vi "PS4000_stream.vi"() -> ()   [LabVIEW 2009]
uses:
  PS4000.dll
  ps4000wrap.dll
  Instance           1 21Saved   PS4000_stream .vi
panel:
  out "Sampling Interval (nanoseconds)":i32
  in  "Number of samples":i32
  in  "Sample Rate (S/s)":u32
  out "bufferLth":i32
  out "Triggered":bool
  in  "Threshold (mV)":i16
  in  "Auto Trigger (ms)":i32 min=1
  in  "Trigger direction":i16(ring) items=["Rising", "Falling"]
  in  "Update settings":bool
  in  "Ch A Coupling":enum32{"Radio Selection 1", "Radio Selection 2"}(radio)
  in  "Ch B Coupling":enum32{"Radio Selection 1", "Radio Selection 2"}(radio)
  out "XY Graph":cluster{"buffer":dbl[], "buffer":dbl[]}(graph)
  in  "Trigger delay (us)":u32
  in  "Ch A Trigger":bool
  in  "A enabled":bool
  in  "B enabled":bool
  out "Channel B":waveform(dbl)(graph)
  in  "Ch B Range":i32(ring) items=["±50 mV", "±100 mV", "±200 mV", "±500 mV", "±1 V", "±2 V", "±5 V", "±10 V", "±20 V", "±50 V", "±100 V"]
  in  "Ch A Range":i32(ring) items=["±50 mV", "±100 mV", "±200 mV", "±500 mV", "±1 V", "±2 V", "±5 V", "±10 V", "±20 V", "±50 V", "±100 V"]
  in  "stop":bool
  out "Channel A":waveform(dbl)(graph)
  # "Streaming example"
  # "(Must be within channel range)"
  # "X-Y Plot"
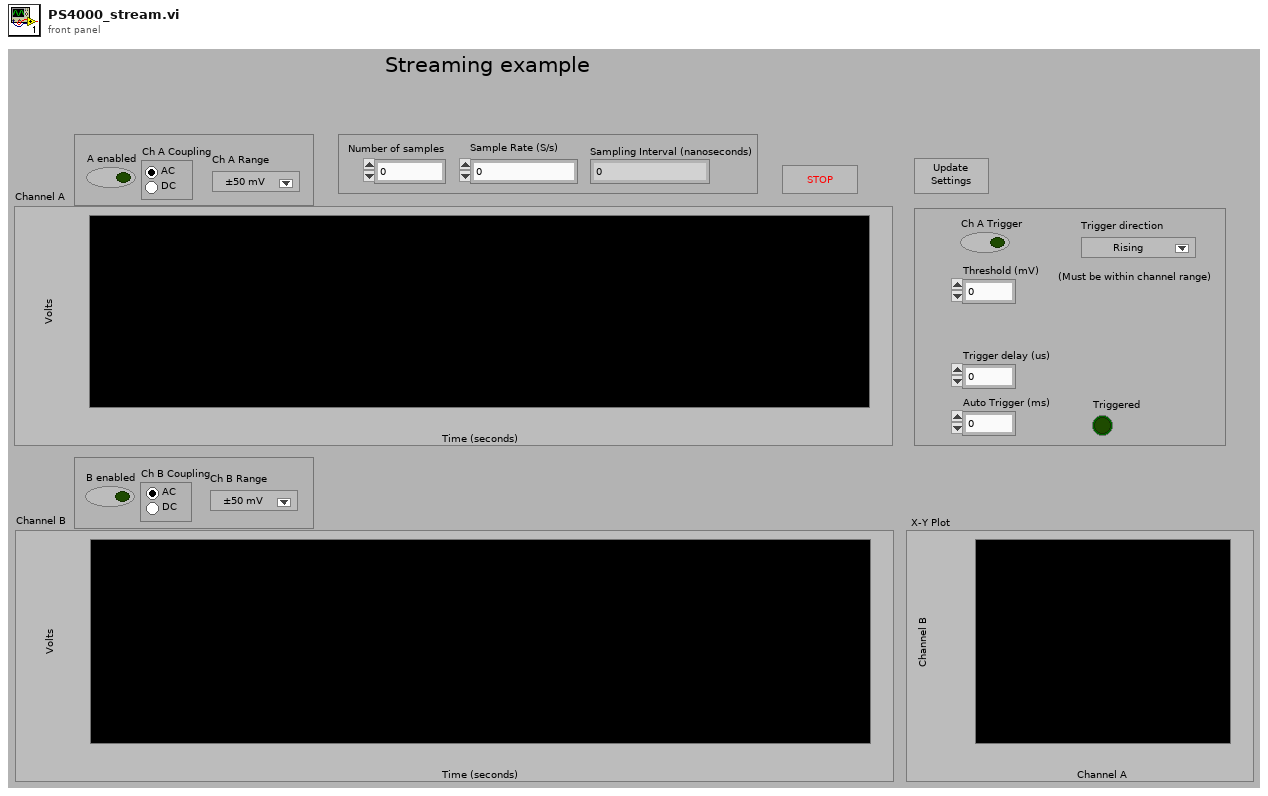
[diagram p1: front panel]
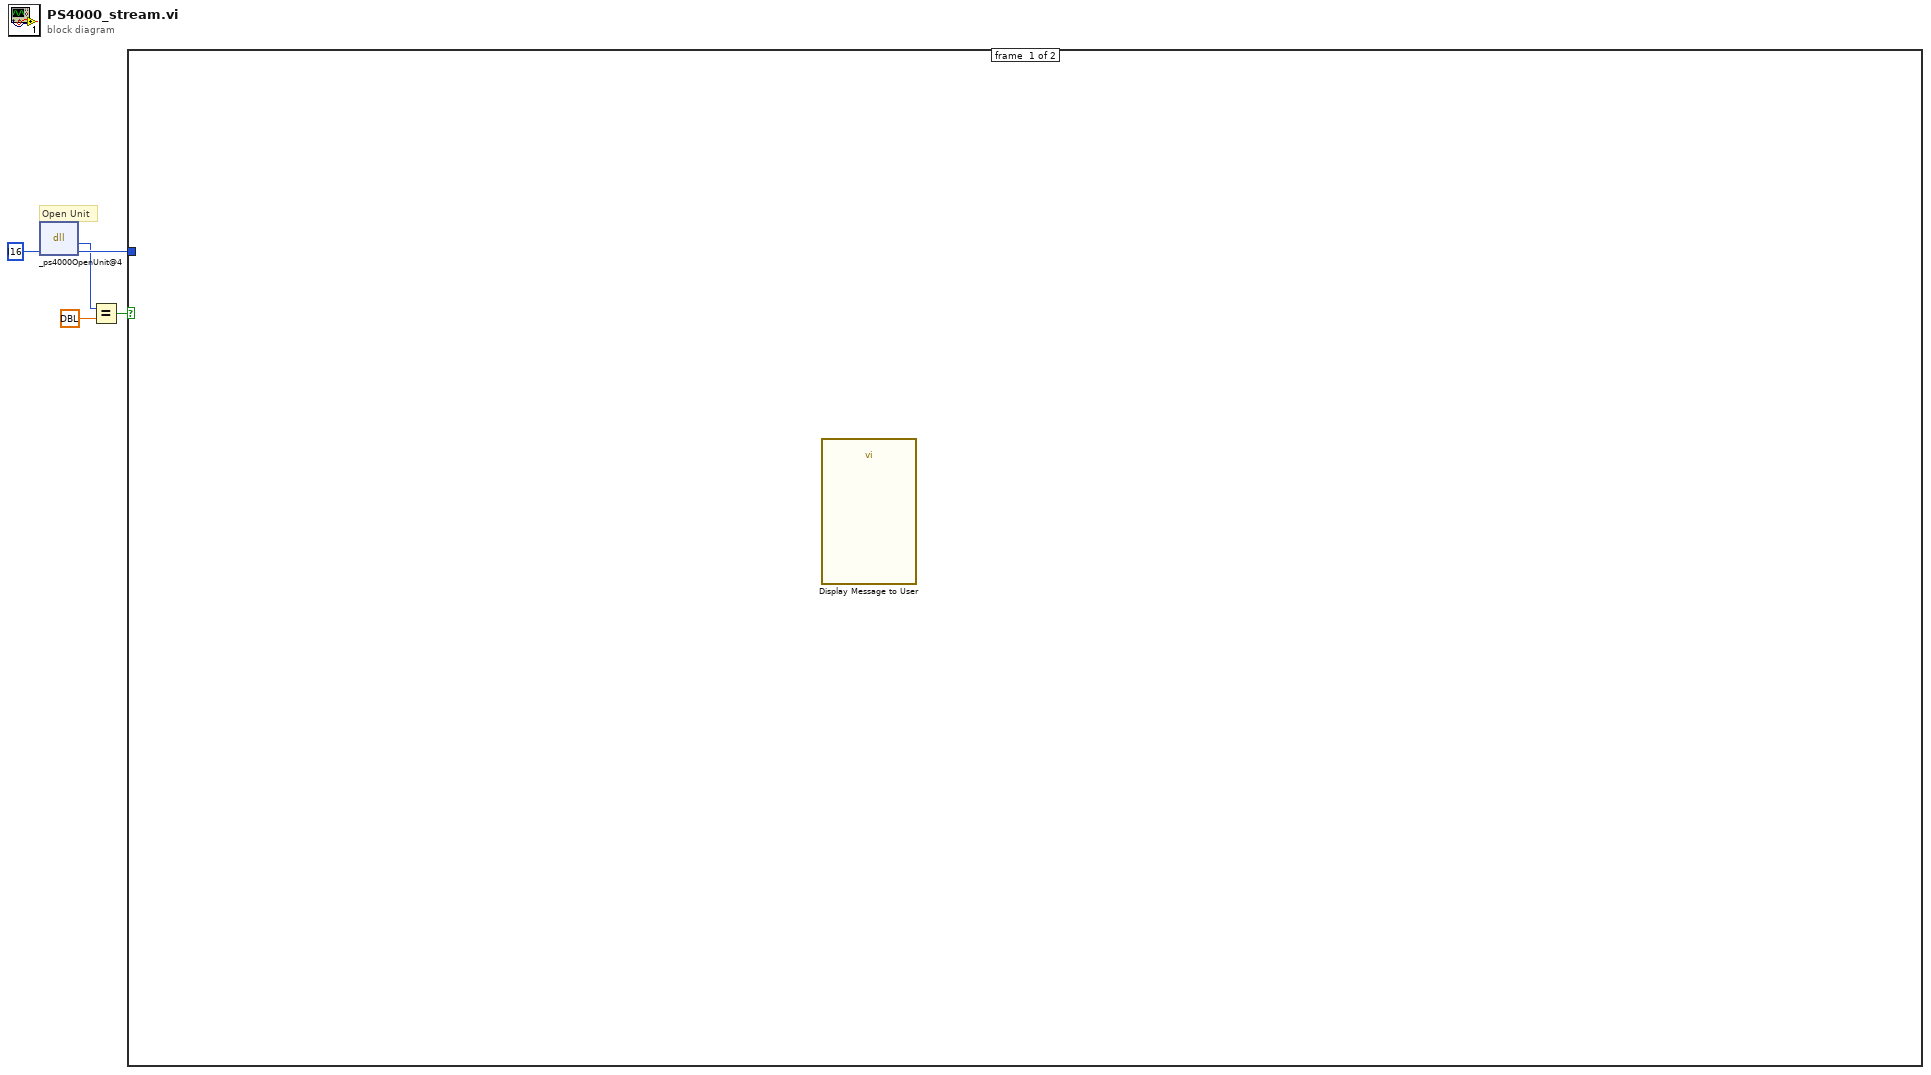
[diagram p0: block diagram]
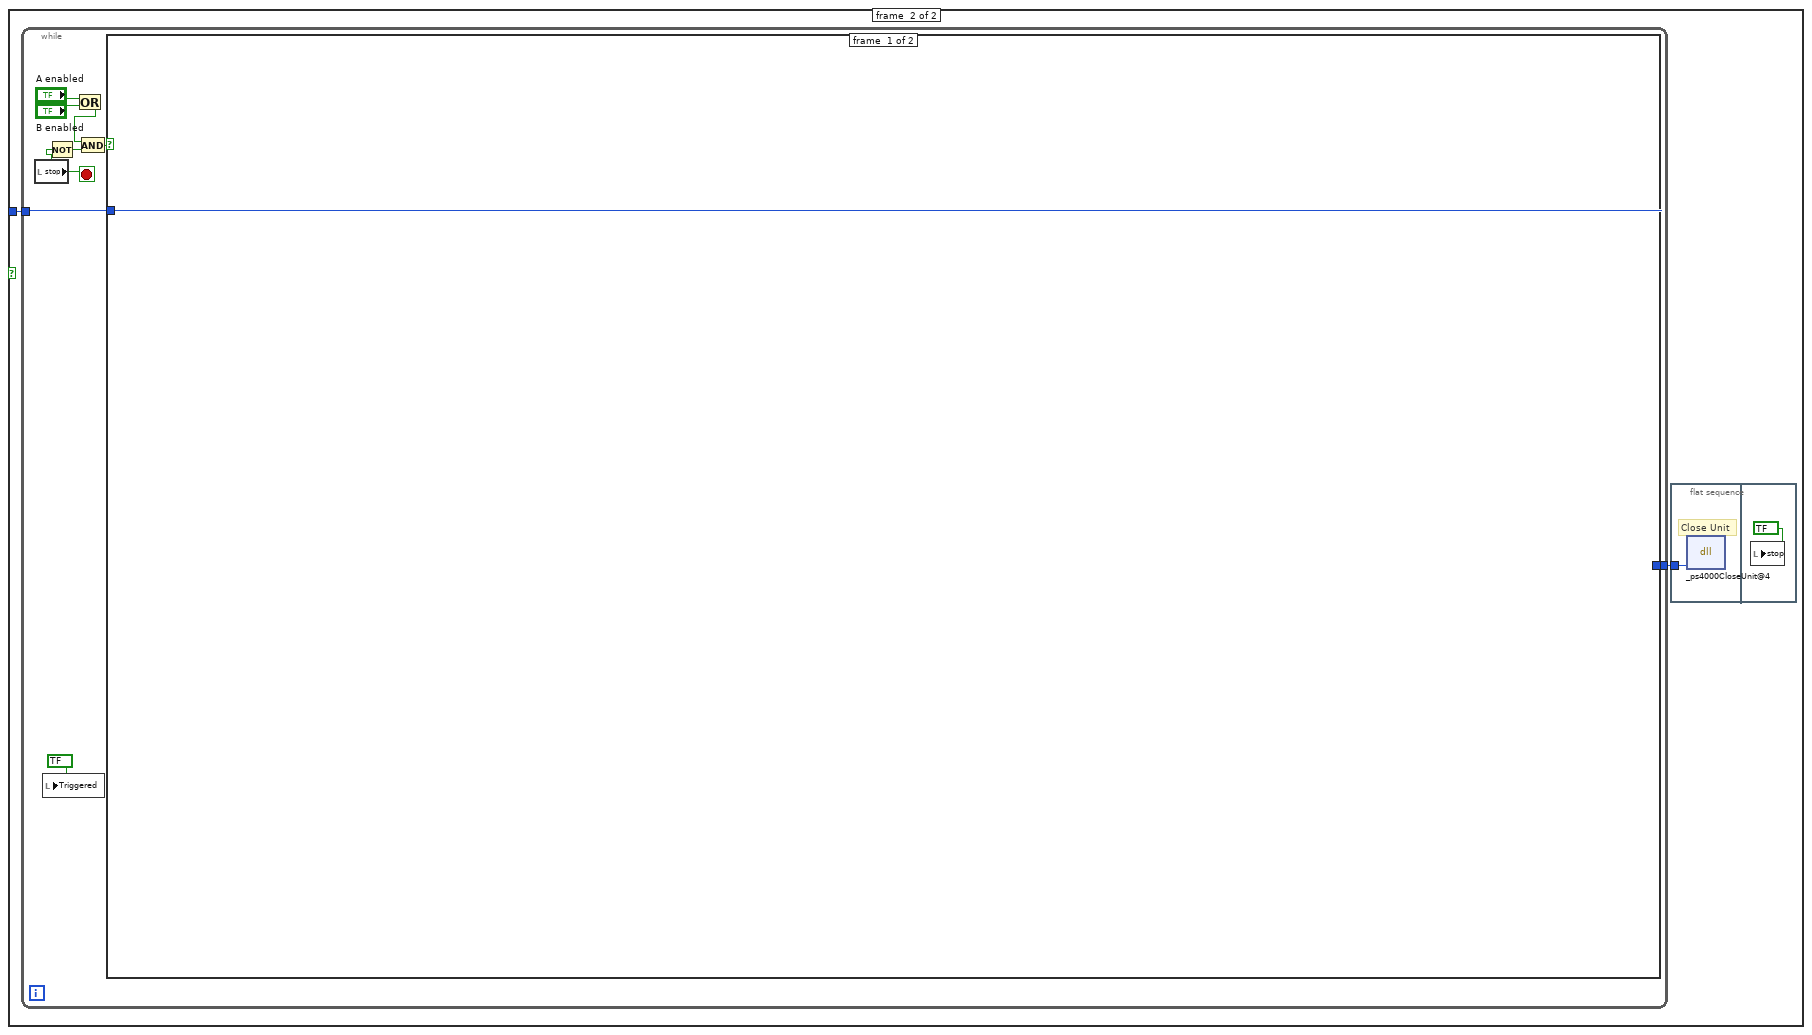
[diagram p2: hidden frame]
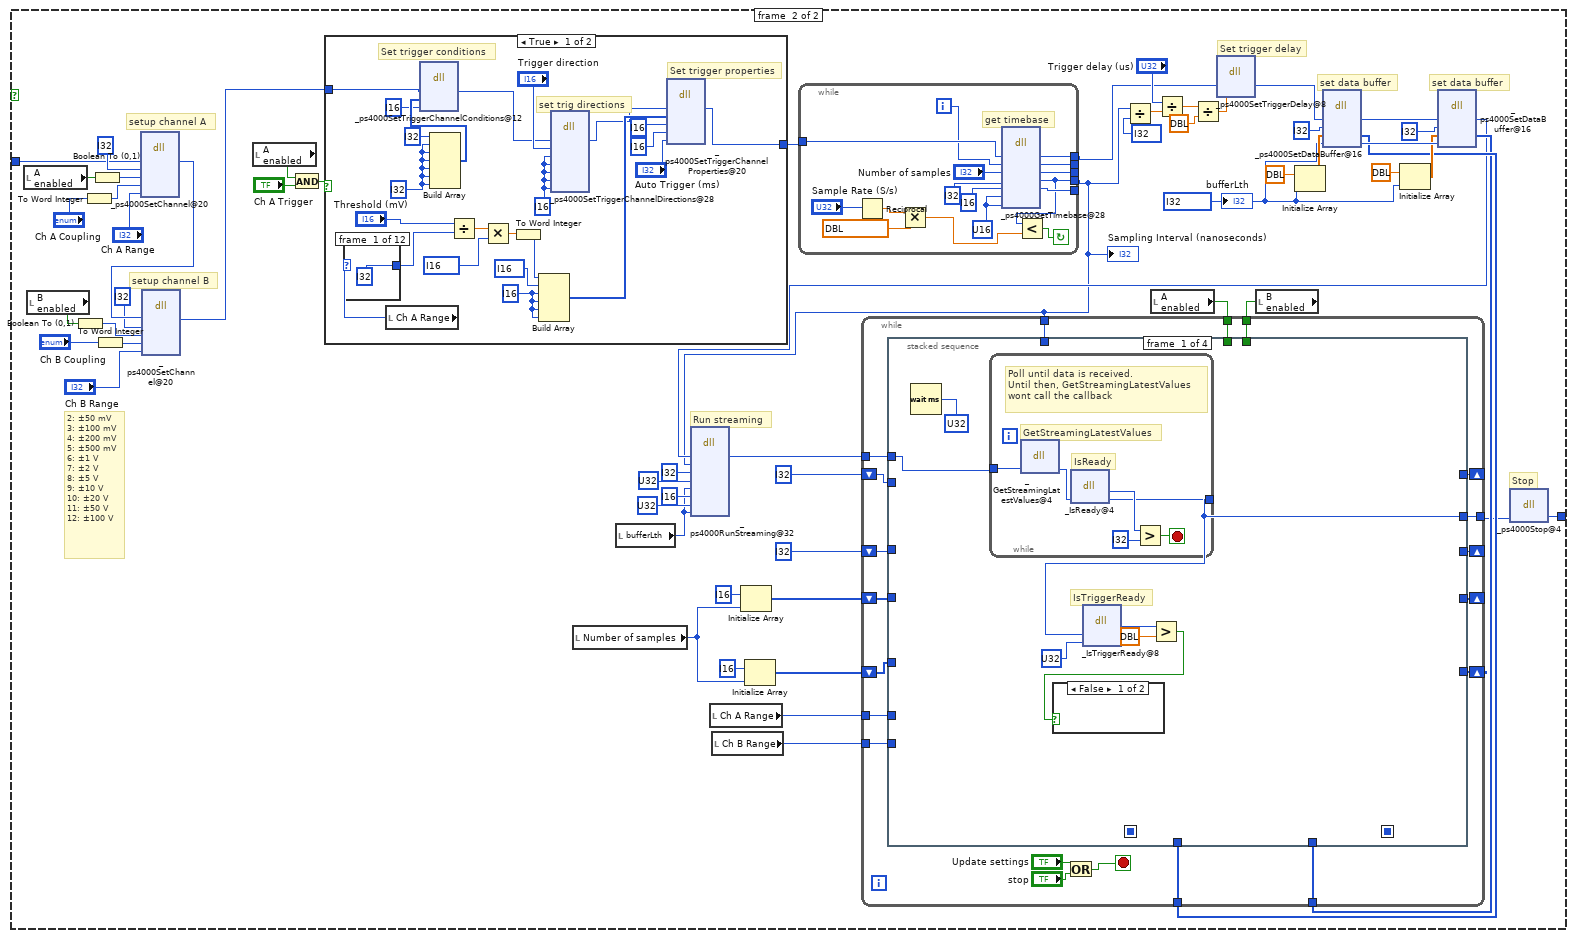
[diagram p3: hidden frame]
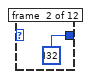
[diagram p4: hidden frame]
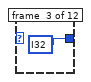
[diagram p5: hidden frame]
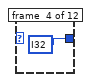
[diagram p6: hidden frame]
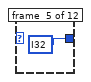
[diagram p7: hidden frame]
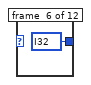
[diagram p8: hidden frame]
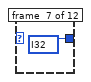
[diagram p9: hidden frame]
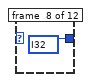
[diagram p10: hidden frame]
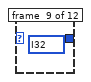
[diagram p11: hidden frame]
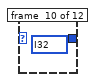
[diagram p12: hidden frame]
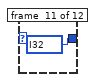
[diagram p13: hidden frame]
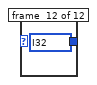
[diagram p14: hidden frame]
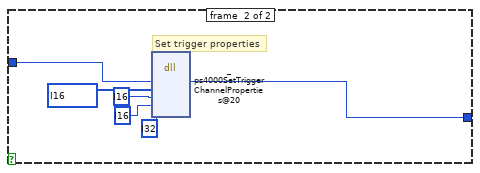
[diagram p15: hidden frame]
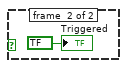
[diagram p16: hidden frame]
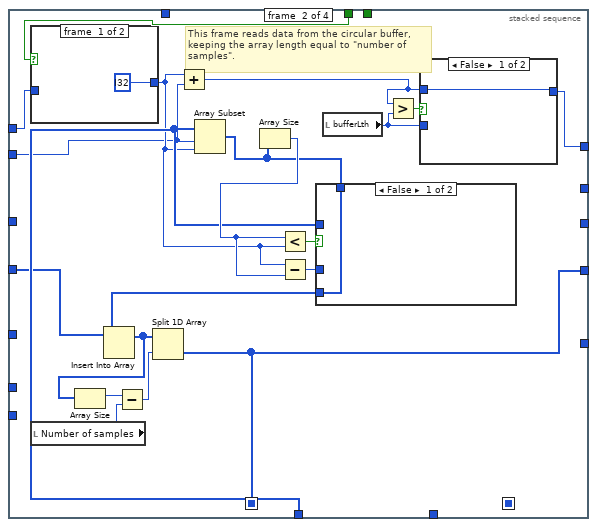
[diagram p17: hidden frame]
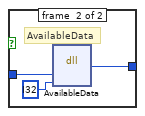
[diagram p18: hidden frame]
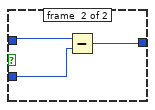
[diagram p19: hidden frame]
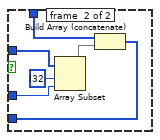
[diagram p20: hidden frame]
diagram:
  # "Open Unit"
  n1 = dll-call lib="PS4000.dll" fn="_ps4000OpenUnit@4" ("ps3000.dll:_ps3000_open_unit@0")("handle"=i16 ?) -> ("PICO_STATUS"=w1:i32, "handle"=w4:i16)  [unwired: 3 in, 2 out]
  n2 = Equal?(x=w1, y=dbl ?) -> (x = y?=w3:bool)
  n3 = case shown="True" w3 {
    tunnel: w4 -> [_ w6]
    frame #0 {
      n4 = call "Display Message to User"() -> ()  [unwired: 10 in, 2 out]
    }
    frame #1 {
      n5 = while {
        tunnel: [w18] -> w7
        tunnel: w6 -> [w15]
        stop <- w10 stop-if-true
        n6 = local read "stop"() -> (w10:bool)
        n7 = local write "Triggered"(bool ? ("triggered?")) -> ()
        n8 = Not(x=w10) -> (.not. x?=w11:bool)
        n9 = Or(x="A enabled", y="B enabled") -> (x .or. y?=w12:bool)
        n10 = And(x=w12, y=w11) -> (x .and. y?=w13:bool)
        n11 = case shown="True" w13 {
          tunnel: [w19 w39] -> w18
          tunnel: w15 -> [w19 w64]
          frame #0 {
          }
          frame #1 {
            w25 = i32 ? ("bufferLth")
            # "Stop"
            # "Run streaming"
            # "Set trigger delay"
            # "setup channel B"
            # "2: ±50 mV\n3: ±100 mV\n4: ±200 mV\n5: ±500 mV\n6: ±1 V\n7: ±2 V\n8: ±5 V\n9: ±10 V\n10: ±20 V\n11: ±50 V\n12: ±100 V"
            # "setup channel A"
            # "set data buffer"
            # "set data buffer"
            n12 = local read "A enabled"() -> (w50:bool)
            n13 = local read "B enabled"() -> (w49:bool)
            n14 = Boolean To (0,1)(Boolean=w49) -> (0, 1=w48:i16)
            n15 = To Word Integer(number="Ch A Coupling") -> (16bit integer=w53:i16)
            n16 = Boolean To (0,1)(Boolean=w50) -> (0, 1=w47:i16)
            n17 = To Word Integer(number="Ch B Coupling") -> (16bit integer=w55:i16)
            n18 = dll-call lib="PS4000.dll" fn="_ps4000SetChannel@20" ("ps3000.dll:_ps3000_open_unit@0")("handle"=w64, "channel"=i32 ?, "enabled"=w47, "dc"=w53, "range"="Ch A Range") -> ("handle"=w68:i16)  [unwired: 8 in, 2 out]
            n19 = dll-call lib="PS4000.dll" fn="_ps4000SetChannel@20" ("ps3000.dll:_ps3000_open_unit@0")("handle"=w68, "channel"=i32 ?, "enabled"=w48, "dc"=w55, "range"="Ch B Range") -> ("handle"=w27:i16)  [unwired: 8 in, 2 out]
            n20 = local read "A enabled"() -> (w56:bool)
            n21 = And(x=w56, y="Ch A Trigger") -> (x .and. y?=w28:bool)
            n22 = case shown="True" w28 {
              tunnel: [w95 w135] -> w22
              tunnel: w27 -> [w97 w130]
              frame #0 {
                w103 = i16 ? ("channelA")
                w106 = i32 ?
                w100 = i16 ? ("element")
                # "set trig directions"
                # "Set trigger conditions"
                # "Set trigger properties"
                n23 = local read "Ch A Range"() -> (w98:i32)
                n24 = case shown="2" w98 {
                  tunnel: [i32 ? i32 ? i32 ? i32 ? i32 ? i32 ? i32 ? i32 ? i32 ? i32 ? i32 ? i32 ?] -> w110
                  frame #0 {
                  }
                  frame #1 {
                  }
                  frame #2 {
                  }
                  frame #3 {
                  }
                  frame #4 {
                  }
                  frame #5 {
                  }
                  frame #6 {
                  }
                  frame #7 {
                  }
                  frame #8 {
                  }
                  frame #9 {
                  }
                  frame #10 {
                  }
                  frame #11 {
                  }
                }
                n25 = Build Array(i32 ? ("element"), w106, w106, w106, w106, w106, w106) -> (w105:i32[])
                n26 = dll-call lib="PS4000.dll" fn="_ps4000SetTriggerChannelConditions@12" ("ps3000.dll:_ps3000_open_unit@0")("handle"=w97, "conditions"=w105, "nConditions"=i16 ?) -> ("handle"=w99:i16)  [unwired: 6 in, 2 out]
                n27 = Divide(x="Threshold (mV)", y=w110) -> (x/y=w112:dbl)
                n28 = Multiply(x=w112, y=i16 ?) -> (x*y=w109:dbl)
                n29 = To Word Integer(number=w109) -> (16bit integer=w108:i16)
                n30 = Build Array(w108, i16 ? ("Minor threshold"), w100, w100, w100, w100) -> (w115:i16[])
                n31 = dll-call lib="PS4000.dll" fn="_ps4000SetTriggerChannelDirections@28" ("ps3000.dll:_ps3000_open_unit@0")("handle"=w99, "channelA"="Trigger direction", "channelB"=w103, "channelC"=w103, "channelD"=w103, "ext"=w103, "aux"=w103) -> ("handle"=w96:i16)  [unwired: 10 in, 2 out]
                n32 = dll-call lib="PS4000.dll" fn="_ps4000SetTriggerChannelProperties@20" ("ps3000.dll:_ps3000_open_unit@0")("handle"=w96, "channelProperties"=w115, "nChannelProperties"=i16 ?, "auxOutputEnable"=i16 ?, "autoTriggerMilliseconds"="Auto Trigger (ms)") -> ("handle"=w95:i16)  [unwired: 8 in, 2 out]
              }
              frame #1 {
                # "Set trigger properties"
                n33 = dll-call lib="PS4000.dll" fn="_ps4000SetTriggerChannelProperties@20" ("ps3000.dll:_ps3000_open_unit@0")("handle"=w130, "channelProperties"=i16[] ?, "nChannelProperties"=i16 ?, "auxOutputEnable"=i16 ?, "autoTriggerMilliseconds"=i32 ?) -> ("handle"=w135:i16)  [unwired: 8 in, 2 out]
              }
            }
            n34 = local read "Number of samples"() -> (w33:i32)
            n35 = local read "bufferLth"() -> (w24:i32)
            n36 = local read "Ch A Range"() -> (w32:i32)
            n37 = local read "Ch B Range"() -> (w31:i32)
            n38 = Initialize Array(i16 ? ("element"), w33) -> (w34:i16[])
            n39 = Initialize Array(i16 ? ("element"), w33) -> (w37:i16[])
            n40 = while {
              tunnel: [w91] -> _
              tunnel: [w90] -> _
              tunnel: [w89] -> w21
              tunnel: [w88] -> _
              tunnel: [w80] -> w20
              tunnel: w22 -> [w87]
              i -> [w85]
              stop <- w81 continue-if-true
              w86 = u16 ? ("segmentIndex")
              # "get timebase"
              n41 = Reciprocal(x="Sample Rate (S/s)") -> (1/x=w83:dbl)
              n42 = Multiply(x=w83, y=dbl ?) -> (x*y=w79:dbl)
              n43 = dll-call lib="PS4000.dll" fn="_ps4000GetTimebase@28" ("ps3000.dll:_ps3000_open_unit@0")("handle"=w87, "timebase"=w85, "noSamples"="Number of samples", "timeIntervalNanoseconds"=i32 ?, "oversample"=i16 ?, "maxSamples"=w86, "segmentIndex"=w86) -> ("handle"=w89:i16, "timebase"=w90:u32, "noSamples"=w88:i32, "timeIntervalNanoseconds"=w80:i32, "oversample"=w91:i16)  [unwired: 6 in, 2 out]
              n44 = Less?(x=w80, y=w79) -> (x < y?=w81:bool)
            }
            "Sampling Interval (nanoseconds)" <- w20
            n45 = Divide(x=w20, y=i32 ? ("x")) -> (x/y=w58:dbl)
            n46 = local read "A enabled"() -> (w30:bool)
            n47 = Divide(x="Trigger delay (us)", y=w58) -> (x/y=w60:dbl)
            n48 = Divide(x=w60, y=dbl ?) -> (x/y=w62:dbl)
            n49 = dll-call lib="PS4000.dll" fn="_ps4000SetTriggerDelay@8" ("ps3000.dll:_ps3000_open_unit@0")("handle"=w21, "delay"=w62) -> ("handle"=w46:i16)  [unwired: 5 in, 2 out]
            n50 = local read "B enabled"() -> (w29:bool)
            n51 = Initialize Array(dbl ? ("element"), w25) -> (w74:dbl[])
            n52 = dll-call lib="PS4000.dll" fn="_ps4000SetDataBuffer@16" ("ps3000.dll:_ps3000_open_unit@0")("handle"=w46, "channel"=i32 ?, "buffer"=w74, "bufferLth"=w25) -> ("handle"=w75:i16, "buffer"=w70:i16[], "bufferLth"=w76:i32)  [unwired: 5 in, 2 out]
            n53 = Initialize Array(dbl ? ("element"), w25) -> (w71:dbl[])
            n54 = dll-call lib="PS4000.dll" fn="_ps4000SetDataBuffer@16" ("ps3000.dll:_ps3000_open_unit@0")("handle"=w75, "channel"=i32 ?, "buffer"=w71, "bufferLth"=w76) -> ("handle"=w26:i16, "buffer"=w69:i16[])  [unwired: 6 in, 2 out]
            n55 = dll-call lib="PS4000.dll" fn="_ps4000RunStreaming@32" ("PS5000.dll:_ps5000RunStreaming@32")("handle"=w26, "sampleInterval"=w20, "sampleIntervalTimeUnits"=i32 ?, "maxPreTriggerSamples"=u32 ?, "maxPostTriggerSamples"=w24, "autoStop"=i16 ?, "downSampleRatio"=u32 ?, "overviewBufferSize"=w24) -> ("handle"=w42:i16)  [unwired: 11 in, 2 out]
            n56 = while {
              tunnel: w70 -> [w155]
              tunnel: w69 -> [w154]
              tunnel: w20 -> [w153]
              tunnel: w42 -> [w152]
              tunnel: [w151] -> w38
              shift-right: [w149] -> _
              shift-left: i32 ? -> [w145]
              shift-right: [w150] -> _
              shift-left: w34 -> [w147]
              shift-right: [w148] -> _
              shift-left: i32 ? -> [w146]
              shift-right: [w144] -> _
              shift-left: w37 -> [w143]
              tunnel: w32 -> [w142]
              tunnel: w31 -> [w141]
              tunnel: w30 -> [w137]
              tunnel: w29 -> [w136]
              stop <- w139 stop-if-true
              n57 = stacked-sequence {
                seq-local: [_ _ w210 _] -> [_ _ _ w245]
                seq-local: [_ w174 _ _] -> [_ _ _ w244]
                tunnel: w155 -> [_ w185 _ _]
                tunnel: w153 -> [_ _ _ w255]
                tunnel: w154 -> [_ _ w207 _]
                tunnel: w152 -> [w157 w179 w216 _]
                tunnel: [w161 _ _ _] -> w151
                tunnel: w147 -> [_ w180 _ _]
                tunnel: [_ w174 _ _] -> w150
                tunnel: w146 -> [_ _ w214 _]
                tunnel: [_ w177 _ _] -> w149
                tunnel: [_ _ w211 _] -> w148
                tunnel: w145 -> [_ w173 _ _]
                tunnel: [_ _ w210 _] -> w144
                tunnel: w143 -> [_ _ w209 _]
                tunnel: w142 -> [_ _ _ w243]
                tunnel: w141 -> [_ _ _ w242]
                tunnel: w137 -> [_ w170 _ w241]
                tunnel: w136 -> [_ _ w205 w240]
                frame #0 {
                  # "IsTriggerReady"
                  n58 = Wait (ms)(milliseconds to wait=u32 ?) -> ()  [unwired: 1 out]
                  n59 = while {
                    tunnel: w157 -> [w165]
                    tunnel: [w164] -> w161
                    stop <- w167 stop-if-true
                    # "GetStreamingLatestValues"
                    # "Poll until data is received. \nUntil then, GetStreamingLatestValues \nwont call the callback"
                    # "IsReady"
                    n60 = dll-call lib="C:/Pico SDK/PS4000sdk_r10_5_0_19/Labview/ps4000wrap.dll" fn="_GetStreamingLatestValues@4" ("PS5000.dll:_ps5000SetDataBuffer@16")("handle"=w165) -> ("handle"=w166:i16)  [unwired: 4 in, 2 out]
                    n61 = dll-call lib="C:/Pico SDK/PS4000sdk_r10_5_0_19/Labview/ps4000wrap.dll" fn="_IsReady@4" ("PS5000.dll:_ps5000SetDataBuffer@16")("handle"=w166) -> ("ready"=w168:i16, "handle"=w164:i16)  [unwired: 3 in, 2 out]
                    n62 = Greater?(x=w168, y=i32 ?) -> (0:w167:bool)
                  }
                  n63 = dll-call lib="C:/Pico SDK/PS4000sdk_r10_5_0_19/Labview/ps4000wrap.dll" fn="_IsTriggerReady@8" ("PS5000.dll:_ps5000SetDataBuffer@16")("handle"=w161, "triggeredAt"=u32 ?) -> ("triggered"=w158:i16)  [unwired: 5 in, 2 out]
                  n64 = Greater?(x=w158, y=dbl ?) -> (0:w160:bool)
                  n65 = case shown="False" w160 {
                    frame #0 {
                    }
                    frame #1 {
                      "Triggered" <- bool ? ("triggered?")
                    }
                  }
                }
                frame #1 {
                  # "This frame reads data from the circular buffer,\nkeeping the array length equal to \"number of\nsamples\"."
                  n66 = case shown="True" w170 {
                    tunnel: w179 -> [_ w193]
                    tunnel: [i32 ? ("numSamples") w192] -> w175
                    frame #0 {
                    }
                    frame #1 {
                      # "AvailableData"
                      n67 = dll-call lib="C:/Pico SDK/PS4000sdk_r10_5_0_19/Labview/ps4000wrap.dll" fn="AvailableData" ("PS5000.dll:_ps5000Stop@4")("handle"=w193, "startIndex"=i32 ?) -> ("numSamples"=w192:u32)  [unwired: 5 in, 2 out]
                    }
                  }
                  n68 = local read "Number of samples"() -> (w172:i32)
                  n69 = Add(x=w175, y=w173) -> (x+y=w176:u32)
                  n70 = Array Subset(array=w185, index=w173, length=w175) -> (w187:i16[])
                  n71 = Array Size(array=w187) -> (size(s)=w189:i32)
                  n72 = Less?(x=w189, y=w175) -> (x < y?=w186:bool)
                  n73 = Subtract(x=w175, y=w189) -> (x-y=w188:u32)
                  n74 = case shown="False" w186 {
                    tunnel: w187 -> [w198 w204]
                    tunnel: [w198 w199] -> w181
                    tunnel: w185 -> [_ w203]
                    tunnel: w188 -> [_ w201]
                    frame #0 {
                    }
                    frame #1 {
                      n75 = Array Subset(array=w203, index=i32 ?, length=w201) -> (w200:i16[])
                      n76 = Build Array (concatenate)(w204, w200) -> (w199:i16[])
                    }
                  }
                  n77 = Insert Into Array(array=w180, new element=w181) -> (w184:i16[])  [unwired: 1 in]
                  n78 = Array Size(array=w184) -> (size(s)=w183:i32)
                  n79 = Subtract(x=w183, y=w172) -> (x-y=w182:i32)
                  n80 = Split 1D Array(array=w184, index=w182) -> (second subarray=w174:i16[])  [unwired: 1 out]
                  n81 = local read "bufferLth"() -> (w171:i32)
                  n82 = Greater?(x=w176, y=w171) -> (0:w178:bool)
                  n83 = case shown="False" w178 {
                    tunnel: [w194 w195] -> w177
                    tunnel: w176 -> [w194 w197]
                    tunnel: w171 -> [_ w196]
                    frame #0 {
                    }
                    frame #1 {
                      n84 = Subtract(x=w197, y=w196) -> (x-y=w195:u32)
                    }
                  }
                }
                frame #2 {
                  # "This frame reads data from the circular buffer,\nkeeping the array length equal to \"number of\nsamples\"."
                  n85 = local read "Number of samples"() -> (w208:i32)
                  n86 = case shown="True" w205 {
                    tunnel: w216 -> [_ w228]
                    tunnel: [i32 ? ("numSamples") w227] -> w212
                    frame #0 {
                    }
                    frame #1 {
                      # "AvailableData"
                      n87 = dll-call lib="C:/Pico SDK/PS4000sdk_r10_5_0_19/Labview/ps4000wrap.dll" fn="AvailableData" ("PS5000.dll:_ps5000Stop@4")("handle"=w228, "startIndex"=i32 ?) -> ("numSamples"=w227:u32)  [unwired: 5 in, 2 out]
                    }
                  }
                  n88 = Add(x=w212, y=w214) -> (x+y=w213:u32)
                  n89 = Array Subset(array=w207, index=w214, length=w212) -> (w222:i16[])
                  n90 = Array Size(array=w222) -> (size(s)=w224:i32)
                  n91 = Less?(x=w224, y=w212) -> (x < y?=w221:bool)
                  n92 = Subtract(x=w212, y=w224) -> (x-y=w223:u32)
                  n93 = local read "bufferLth"() -> (w206:i32)
                  n94 = case shown="False" w221 {
                    tunnel: w222 -> [w233 w239]
                    tunnel: [w233 w234] -> w217
                    tunnel: w207 -> [_ w238]
                    tunnel: w223 -> [_ w236]
                    frame #0 {
                    }
                    frame #1 {
                      n95 = Array Subset(array=w238, index=i32 ?, length=w236) -> (w235:i16[])
                      n96 = Build Array (concatenate)(w239, w235) -> (w234:i16[])
                    }
                  }
                  n97 = Insert Into Array(array=w209, new element=w217) -> (w220:i16[])  [unwired: 1 in]
                  n98 = Array Size(array=w220) -> (size(s)=w219:i32)
                  n99 = Subtract(x=w219, y=w208) -> (x-y=w218:i32)
                  n100 = Split 1D Array(array=w220, index=w218) -> (second subarray=w210:i16[])  [unwired: 1 out]
                  n101 = Greater?(x=w213, y=w206) -> (0:w215:bool)
                  n102 = case shown="False" w215 {
                    tunnel: [w229 w230] -> w211
                    tunnel: w213 -> [w229 w232]
                    tunnel: w206 -> [_ w231]
                    frame #0 {
                    }
                    frame #1 {
                      n103 = Subtract(x=w232, y=w231) -> (x-y=w230:u32)
                    }
                  }
                }
                frame #3 {
                  n104 = Divide(x=w255, y=i32 ?) -> (x/y=w253:dbl)
                  n105 = case shown="Default" w243 {
                    tunnel: w244 -> [w316 w320 w325 w328 w332 w338 w343 w348 w353 w358 w363 w368]
                    tunnel: [w316 w318 w323 w327 w333 w337 w342 w347 w352 w357 w362 w367] -> w248
                    frame #0 {
                    }
                    frame #1 {
                      n106 = Multiply(x=dbl ?, y=w320) -> (x*y=w319:dbl[])
                      n107 = Divide(x=w319, y=i32 ?) -> (x/y=w318:dbl[])
                    }
                    frame #2 {
                      n108 = Multiply(x=dbl ?, y=w325) -> (x*y=w324:dbl[])
                      n109 = Divide(x=w324, y=i32 ?) -> (x/y=w323:dbl[])
                    }
                    frame #3 {
                      n110 = Multiply(x=dbl ?, y=w328) -> (x*y=w330:dbl[])
                      n111 = Divide(x=w330, y=i32 ?) -> (x/y=w327:dbl[])
                    }
                    frame #4 {
                      n112 = Multiply(x=dbl ?, y=w332) -> (x*y=w335:dbl[])
                      n113 = Divide(x=w335, y=i32 ?) -> (x/y=w333:dbl[])
                    }
                    frame #5 {
                      n114 = Multiply(x=dbl ?, y=w338) -> (x*y=w340:dbl[])
                      n115 = Divide(x=w340, y=i32 ?) -> (x/y=w337:dbl[])
                    }
                    frame #6 {
                      n116 = Multiply(x=dbl ?, y=w343) -> (x*y=w345:dbl[])
                      n117 = Divide(x=w345, y=i32 ?) -> (x/y=w342:dbl[])
                    }
                    frame #7 {
                      n118 = Multiply(x=dbl ?, y=w348) -> (x*y=w350:dbl[])
                      n119 = Divide(x=w350, y=i32 ?) -> (x/y=w347:dbl[])
                    }
                    frame #8 {
                      n120 = Multiply(x=dbl ?, y=w353) -> (x*y=w355:dbl[])
                      n121 = Divide(x=w355, y=i32 ?) -> (x/y=w352:dbl[])
                    }
                    frame #9 {
                      n122 = Multiply(x=dbl ?, y=w358) -> (x*y=w360:dbl[])
                      n123 = Divide(x=w360, y=i32 ?) -> (x/y=w357:dbl[])
                    }
                    frame #10 {
                      n124 = Multiply(x=dbl ?, y=w363) -> (x*y=w365:dbl[])
                      n125 = Divide(x=w365, y=i32 ?) -> (x/y=w362:dbl[])
                    }
                    frame #11 {
                      n126 = Multiply(x=dbl ?, y=w368) -> (x*y=w370:dbl[])
                      n127 = Divide(x=w370, y=i32 ?) -> (x/y=w367:dbl[])
                    }
                  }
                  n128 = Get Date/Time In Seconds() -> (seconds since 1Jan1904=w252:timestamp)
                  n129 = Bundle By Name("t0"=w252, "dt"=w253, "Y"=w248) -> (→"Channel A":waveform(dbl))  [unwired: 1 in]
                  n130 = case shown="6" w242 {
                    tunnel: w245 -> [w260 w264 w269 w272 w276 w282 w287 w292 w297 w302 w307 w312]
                    tunnel: [w260 w262 w267 w271 w277 w281 w286 w291 w296 w301 w306 w311] -> w249
                    frame #0 {
                    }
                    frame #1 {
                      n131 = Multiply(x=dbl ?, y=w264) -> (x*y=w263:dbl[])
                      n132 = Divide(x=w263, y=i32 ?) -> (x/y=w262:dbl[])
                    }
                    frame #2 {
                      n133 = Multiply(x=dbl ?, y=w269) -> (x*y=w268:dbl[])
                      n134 = Divide(x=w268, y=i32 ?) -> (x/y=w267:dbl[])
                    }
                    frame #3 {
                      n135 = Multiply(x=dbl ?, y=w272) -> (x*y=w274:dbl[])
                      n136 = Divide(x=w274, y=i32 ?) -> (x/y=w271:dbl[])
                    }
                    frame #4 {
                      n137 = Multiply(x=dbl ?, y=w276) -> (x*y=w279:dbl[])
                      n138 = Divide(x=w279, y=i32 ?) -> (x/y=w277:dbl[])
                    }
                    frame #5 {
                      n139 = Multiply(x=dbl ?, y=w282) -> (x*y=w284:dbl[])
                      n140 = Divide(x=w284, y=i32 ?) -> (x/y=w281:dbl[])
                    }
                    frame #6 {
                      n141 = Multiply(x=dbl ?, y=w287) -> (x*y=w289:dbl[])
                      n142 = Divide(x=w289, y=i32 ?) -> (x/y=w286:dbl[])
                    }
                    frame #7 {
                      n143 = Multiply(x=dbl ?, y=w292) -> (x*y=w294:dbl[])
                      n144 = Divide(x=w294, y=i32 ?) -> (x/y=w291:dbl[])
                    }
                    frame #8 {
                      n145 = Multiply(x=dbl ?, y=w297) -> (x*y=w299:dbl[])
                      n146 = Divide(x=w299, y=i32 ?) -> (x/y=w296:dbl[])
                    }
                    frame #9 {
                      n147 = Multiply(x=dbl ?, y=w302) -> (x*y=w304:dbl[])
                      n148 = Divide(x=w304, y=i32 ?) -> (x/y=w301:dbl[])
                    }
                    frame #10 {
                      n149 = Multiply(x=dbl ?, y=w307) -> (x*y=w309:dbl[])
                      n150 = Divide(x=w309, y=i32 ?) -> (x/y=w306:dbl[])
                    }
                    frame #11 {
                      n151 = Multiply(x=dbl ?, y=w312) -> (x*y=w314:dbl[])
                      n152 = Divide(x=w314, y=i32 ?) -> (x/y=w311:dbl[])
                    }
                  }
                  n153 = Bundle By Name("t0"=w252, "dt"=w253, "Y"=w249) -> (→"Channel B":waveform(dbl))  [unwired: 1 in]
                  n154 = And(x=w240, y=w241) -> (x .and. y?=w247:bool)
                  n155 = case shown="True" w247 {
                    tunnel: w249 -> [_ w259]
                    tunnel: w248 -> [_ w258]
                    tunnel: [cluster{"buffer":dbl[], "buffer":dbl[]} ? w257] -> w246
                    frame #0 {
                    }
                    frame #1 {
                      n156 = Bundle(w258, w259) -> (w257:cluster{dbl[], dbl[]})  [unwired: 1 in]
                    }
                  }
                  "XY Graph" <- w246
                }
              }
              n157 = Or(x="Update settings", y="stop") -> (x .or. y?=w139:bool)
            }
            n158 = dll-call lib="PS4000.dll" fn="_ps4000Stop@4" ("PS5000.dll:_ps5000Stop@4")("handle"=w38) -> ("handle"=w39:i16)  [unwired: 4 in, 2 out]
            "bufferLth" <- w25
          }
        }
      }
      n159 = flat-sequence {
        tunnel: w7 -> [w8]
        frame #0 {
          # "Close Unit"
          n160 = dll-call lib="PS4000.dll" fn="_ps4000CloseUnit@4" ("ps3000.dll:_ps3000_open_unit@0")("handle"=w8) -> ()  [unwired: 5 in, 2 out]
        }
        frame #1 {
          n161 = local write "stop"(bool ? ("stop")) -> ()
        }
      }
    }
  }
